vi "Workspace - Load.vi"(7 "This VI":refnum<vi>, 8 "error in":errorcluster, 10 "VI Refs":refnum<vi>[](array[refnum]), 11 "Subhost Names":string[](array[string])) -> (0 "error out":errorcluster, 1 "PanelSubhost":i32, 2 "VI Refs out":refnum<vi>[](array[refnum]), 3 "Subhost Names out":string[](array[string]), 5 "_Subhost-FP.DockStates":bool[](array[boolean]))   [LabVIEW 2016]
uses:
  <vilib>/Utility/miscctls.llb/LVRectTypeDef.ctl
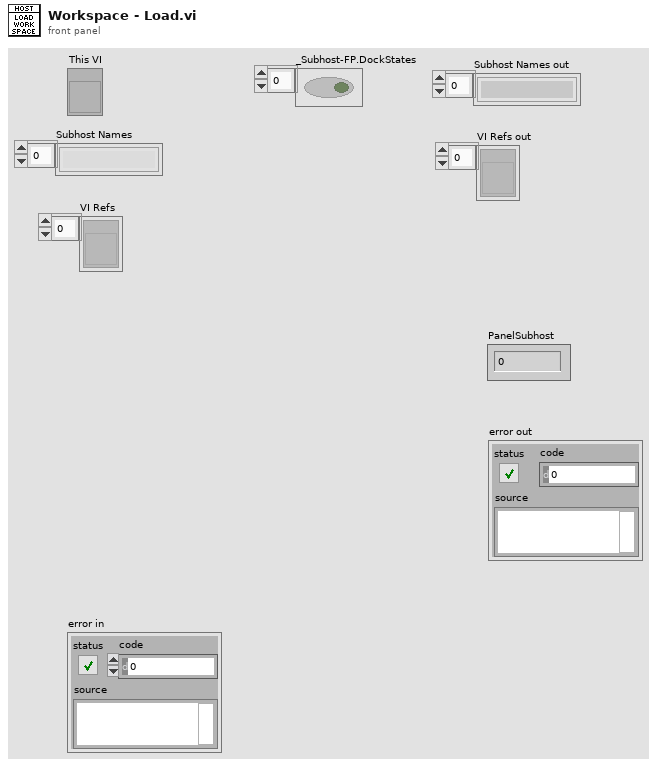
[diagram p1: front panel]
types:
  T1 = typedef "LVRectTypeDef.ctl" = cluster{"Left":i16, "Top":i16, "Right":i16, "Bottom":i16}
  T2 = cluster{"Display Name":string, "Front Panel.WinBounds":T1, "FP.State":enum32{"Invalid", "Standard", "Closed", "Hidden", "Minimized", "Maximized"}, "FP.Monitor":u16, "Boolean":bool}[]
  T3 = enum16{"open", "replace", "create", "open or create", "replace or create", "replace or create with confirmation"}
  T4 = cluster{"Display Name":string, "Front Panel.WinBounds":T1, "FP.State":enum32{"Invalid", "Standard", "Closed", "Hidden", "Minimized", "Maximized"}, "FP.Monitor":u16, "Boolean":bool}
  T5 = enum32{"Invalid", "Standard", "Closed", "Hidden", "Minimized", "Maximized"}
  T6 = typedef "LVPointTypeDef.ctl" = cluster{"Horizontal":i16, "Vertical":i16}
  T7 = typedef "LVAllMonitorsDisplayTypeDef.ctl" = cluster{"Bounds":cluster{"Left":i16, "Top":i16, "Right":i16, "Bottom":i16}, "Depth":i16}[]
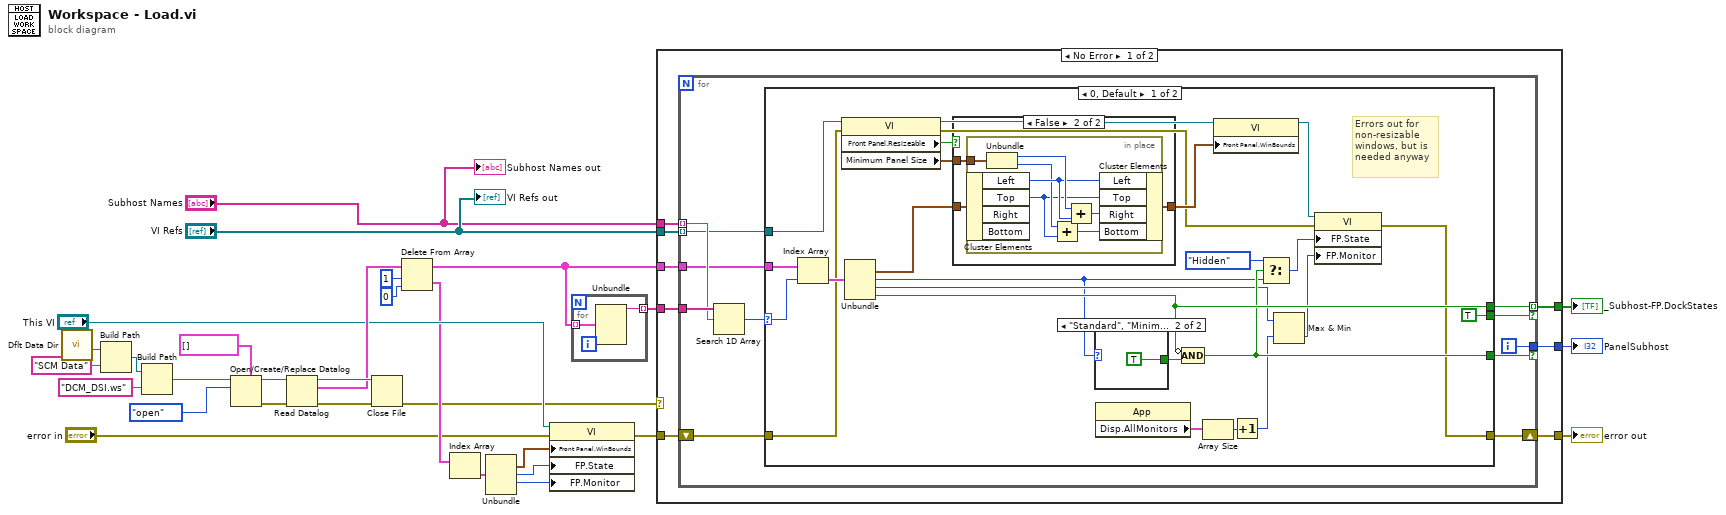
[diagram p0: block diagram]
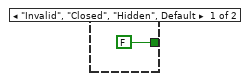
[diagram p3: hidden frame]
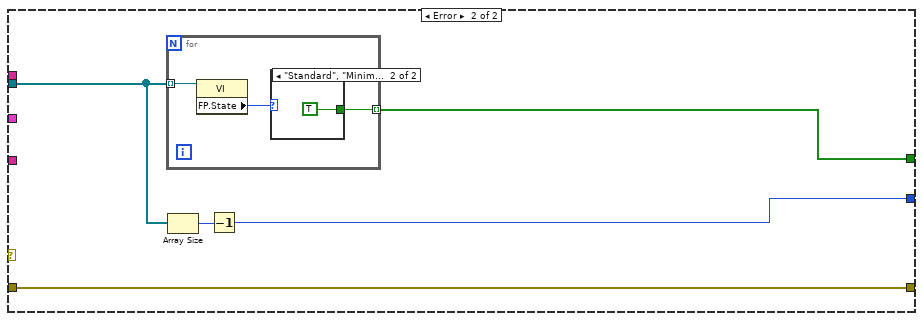
[diagram p5: hidden frame]
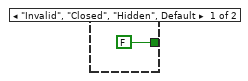
[diagram p6: hidden frame]
diagram:
  n1 = call <vilib>:"Dflt Data Dir.vi"() -> ("App:Default Data Directory"=w3:path)
  n2 = Build Path(base path=w3, name or relative path="SCM Data") -> (appended path=w1:path)
  n3 = Build Path(base path=w1, name or relative path="DCM_DSI.ws") -> (appended path=w26:path)
  n4 = Open/Create/Replace Datalog(5:T2 [] ("Array"), 10:T3."open" ("operation (0:open)"), 11:w26) -> (0:w24:errorcluster, 3:w28:refnum<k1>)  [unwired: 3 in, 1 out]
  n5 = Read Datalog(4:w24, 7:w28) -> (0:w30:errorcluster, 2:w19:T2, 3:w29:refnum<k1>)  [unwired: 1 in]
  n6 = Close File(refnum=w29, error in=w30) -> (error out=w4:errorcluster)  [unwired: 1 out]
  n7 = Delete From Array(array=w19, length=1, index=0) -> (deleted portion=w14:T2, array with subset deleted=w18:T2)
  n8 = Index Array(array=w14) -> (element=w13:T4)  [unwired: 1 in]
  n9 = Unbundle(w13) -> ("Front Panel.WinBounds"=w12:T1, "FP.State"=w11:T5, "FP.Monitor"=w10:u16)  [unwired: 2 out]
  n10 = property class="VI"(reference="This VI", error in="error in", "Front Panel.WinBounds"=w12, "FP.State"=w11, "FP.Monitor"=w10) -> (error out=w8:errorcluster)  [unwired: 1 out]
  n11 = for {
    tunnel: w18 -> [w32] mode=indexing
    tunnel: [w31] -> w22 mode=indexing
    n12 = Unbundle(w32) -> ("Display Name"=w31:string)  [unwired: 4 out]
  }
  n13 = case shown="No Error" w4 {
    tunnel: "VI Refs" -> [w40 w94]
    tunnel: "Subhost Names" -> [w39 _]
    tunnel: w22 -> [w38 _]
    tunnel: w18 -> [w37 _]
    tunnel: [w36 w95] -> w21
    tunnel: [w35 w92] -> w20
    tunnel: [w34 w91] -> w7
    tunnel: w8 -> [w33 w91]
    frame No Error {
      n14 = for {
        tunnel: w40 -> [w48] mode=indexing
        tunnel: w39 -> [w50] mode=indexing
        shift-right: [w42] -> w34
        shift-left: w33 -> [w41]
        tunnel: w38 -> [w51]
        tunnel: w37 -> [w49]
        tunnel: [w46] -> w36 mode=indexing if=w44
        tunnel: [w43] -> w35 if=w45
        i -> [w43]
        n15 = Search 1D Array(1D array=w51, element=w50) -> (index of element=w47:i32)  [unwired: 1 in]
        n16 = case shown="0, Default" w47 {
          selector: w47 -> [w74 _]
          tunnel: w49 -> [w76 _]
          tunnel: w48 -> [w57 _]
          tunnel: [w71 _] -> w46
          tunnel: [TRUE _] -> w44
          tunnel: w41 -> [w61 w90]
          tunnel: [w60 w90] -> w42
          tunnel: [w68 _] -> w45
          frame 0, Default {
            # "Errors out for\nnon-resizable\nwindows, but is\nneeded anyway"
            n17 = Index Array(array=w76, index=w74) -> (element=w75:T4)
            n18 = property class="VI"(reference=w57, error in=w61) -> (reference out=w54:refnum<vi>, error out=w53:errorcluster, "Front Panel.Resizeable"=w59:bool, "Minimum Panel Size"=w52:T6)
            n19 = Unbundle(w75) -> ("Front Panel.WinBounds"=w58:T1, "FP.State"=w65:T5, "FP.Monitor"=w66:u16, "Boolean"=w71:bool)  [unwired: 1 out]
            n20 = case shown="False" w59 {
              tunnel: w58 -> [w77 w80]
              tunnel: [w77 w79] -> w55
              tunnel: w52 -> [_ w78]
              frame True {
              }
              frame False {
                n21 = in-place {
                  in-place-border: w78 -> [w87]
                  n22 = in-place-cluster #1(w80) -> ("Left"=w85:i16, "Top"=w82:i16)  [unwired: 2 out]
                  n23 = Unbundle(w87) -> ("Horizontal"=w86:i16, "Vertical"=w83:i16)
                  n24 = Add(x=w83, y=w82) -> (x+y=w81:i16)
                  n25 = Add(x=w86, y=w85) -> (x+y=w84:i16)
                  n26 = in-place-cluster #1("Left"=w85, "Top"=w82, "Right"=w84, "Bottom"=w81) -> (w79:T1)
                }
              }
            }
            n27 = case shown="\"Standard\", \"Minimized\", \"Maximized\"" w65 {
              tunnel: [FALSE TRUE] -> w72
              frame "Invalid", "Closed", "Hidden", Default {
              }
              frame "Standard", "Minimized", "Maximized" {
              }
            }
            n28 = property class="App"() -> ("Disp.AllMonitors"=w70:T7)  [unwired: 2 in, 2 out]
            n29 = Compound Arithmetic op=AND(invert w71, w72) -> (w68:bool)
            n30 = Array Size(array=w70) -> (size(s)=w69:i32)
            n31 = property class="VI"(reference=w54, "Front Panel.WinBounds"=w55) -> (reference out=w56:refnum<vi>)  [unwired: 1 in, 1 out]
            n32 = Increment(x=w69) -> (x+1=w64:i32)
            n33 = Select(t=T5."Hidden" ("Front Panel Window:State"), s=w68, f=w65) -> (s? t:f=w63:T5)
            n34 = Max & Min(x=w66, y=w64) -> (min(x,y)=w62:i32)  [unwired: 1 out]
            n35 = property class="VI"(reference=w56, error in=w53, "FP.State"=w63, "FP.Monitor"=w62) -> (error out=w60:errorcluster)  [unwired: 1 out]
          }
          frame -1 {
          }
        }
      }
    }
    frame Error {
      n36 = for {
        tunnel: w94 -> [w98] mode=indexing
        tunnel: [w96] -> w95 mode=indexing
        n37 = property class="VI"(reference=w98) -> ("FP.State"=w97:T5)  [unwired: 1 in, 2 out]
        n38 = case shown="\"Standard\", \"Minimized\", \"Maximized\"" w97 {
          tunnel: [FALSE TRUE] -> w96
          frame "Invalid", "Closed", "Hidden", Default {
          }
          frame "Standard", "Minimized", "Maximized" {
          }
        }
      }
      n39 = Array Size(array=w94) -> (size(s)=w93:i32)
      n40 = Decrement(x=w93) -> (x-1=w92:i32)
    }
  }
  "_Subhost-FP.DockStates" <- w21
  "PanelSubhost" <- w20
  "error out" <- w7
  "Subhost Names out" <- "Subhost Names"
  "VI Refs out" <- "VI Refs"
